vi "all physical channels.vi"() -> ()   [LabVIEW 2018]
uses:
  <resource>/objmgr/daqmx.rc
panel:
  out "Array":tag[][](array[tag])
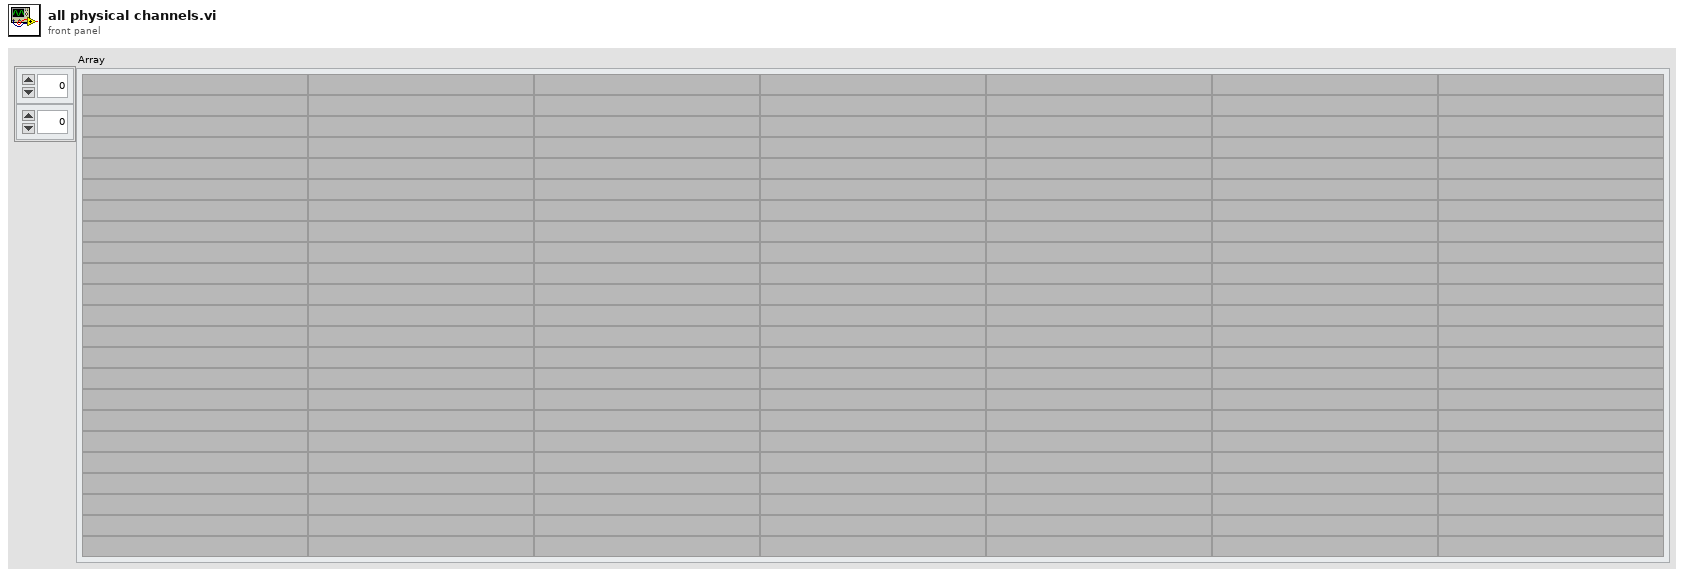
[diagram p1: front panel]
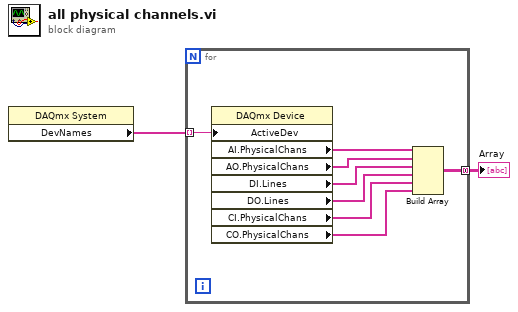
[diagram p0: block diagram]
diagram:
  n1 = property class="DAQmx System"() -> ("DevNames"=w2:tag[])  [unwired: 2 in, 2 out]
  n2 = for {
    tunnel: w2 -> [w10] mode=indexing
    tunnel: [w3] -> w1 mode=concatenating
    n3 = property class="DAQmx Device"("ActiveDev"=w10) -> ("AI.PhysicalChans"=w9:tag[], "AO.PhysicalChans"=w8:tag[], "DI.Lines"=w7:tag[], "DO.Lines"=w6:tag[], "CI.PhysicalChans"=w5:tag[], "CO.PhysicalChans"=w4:tag[])  [unwired: 2 in, 2 out]
    n4 = Build Array(w9, w8, w7, w6, w5, w4) -> (w3:tag[][])
  }
  "Array" <- w1
